vi "Actor Tracker.vi"(8 "error in":errorcluster, 10 "Context":T1, 11 "_Parent Actor Template in":refnum<class "_Parent Actor Template.lvclass">) -> (0 "error out":errorcluster, 3 "_Parent Actor Template out":refnum<class "_Parent Actor Template.lvclass">)   [LabVIEW 2016, in "_Parent Actor Template.lvlib" / "_Parent Actor Template.lvclass"]
uses:
  _Parent Actor Template.lvclass
  Enum - Debug Context.ctl
panel:
  out "Still Running":i32(listbox)
  out "Shutdown\nComplete":bool
  out "Stopped":i32
  out "Started":i32
  out "Shutdown":i32(listbox)
  out "Startup":i32(listbox)
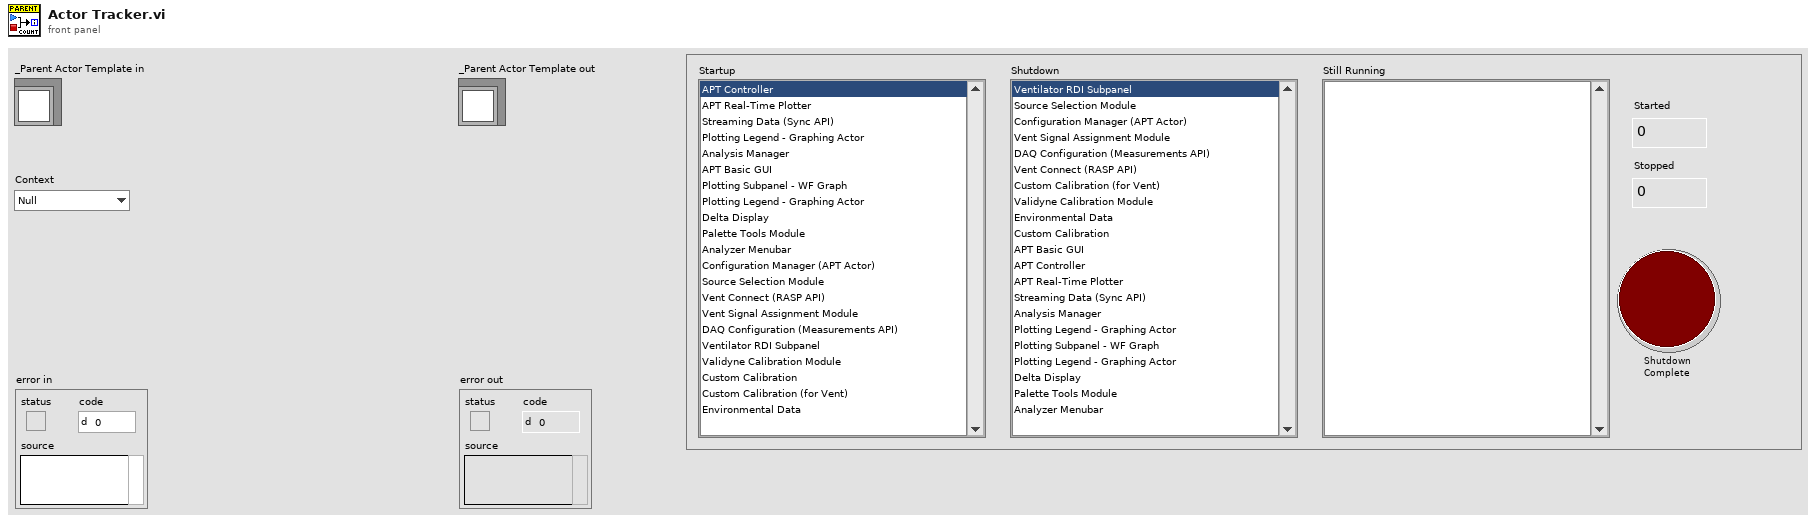
[diagram p1: front panel]
types:
  T1 = typedef "_Parent Actor Template.lvlib/_Parent Actor Template.lvclass/Enum - Debug Context.ctl" = enum16{"Null", "Startup", "Shutdown"}
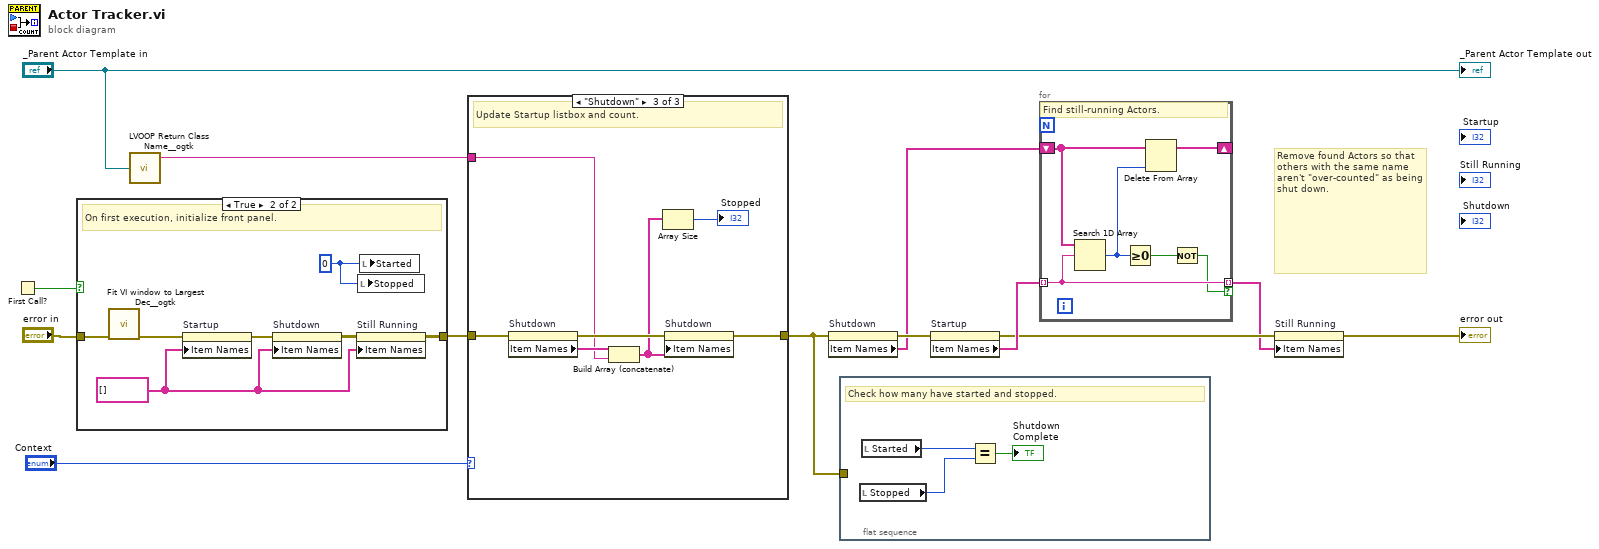
[diagram p0: block diagram]
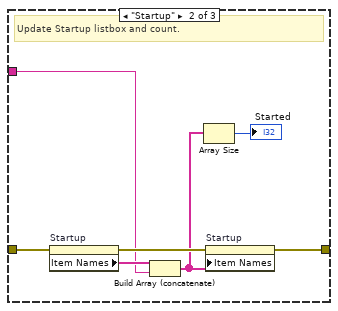
[diagram p3: hidden frame]
diagram:
  # "Remove found Actors so that others with the same name aren't \"over-counted\" as being shut down."
  n1 = First Call?() -> (First Call?: T/F=w12:bool)
  n2 = case shown="True" w12 {
    tunnel: "error in" -> [w14 w21]
    tunnel: [w14 w17] -> w9
    frame False {
    }
    frame True {
      w15 = 0 ("Started")
      w16 = string[] [] ("Item Names")
      # "On first execution, initialize front panel."
      n3 = call <userlib>:"Fit VI window to Largest Dec__ogtk.vi"("error in (no error)"=w21) -> ("error out"=w18:errorcluster)  [unwired: 5 in, 1 out]
      n4 = property on="Startup" class="LstBox (strict)"(error in=w18, "Item Names"=w16) -> (error out=w20:errorcluster)  [unwired: 1 in, 1 out]
      n5 = property on="Shutdown" class="LstBox (strict)"(error in=w20, "Item Names"=w16) -> (error out=w19:errorcluster)  [unwired: 1 in, 1 out]
      n6 = property on="Still Running" class="LstBox (strict)"(error in=w19, "Item Names"=w16) -> (error out=w17:errorcluster)  [unwired: 1 in, 1 out]
      n7 = local write "Stopped"(w15) -> ()
      n8 = local write "Started"(w15) -> ()
    }
  }
  n9 = call <userlib>:"LVOOP Return Class Name__ogtk.vi"("Object"="_Parent Actor Template in") -> ("Class Base Name"=w8:string)  [unwired: 2 out]
  n10 = case shown="\"Shutdown\"" "Context" {
    tunnel: [w22 w27 w34] -> w1
    tunnel: w9 -> [w22 w29 w36]
    tunnel: w8 -> [_ w25 w32]
    frame "Null", Default {
    }
    frame "Startup" {
      # "Update Startup listbox and count."
      n11 = property on="Startup" class="LstBox (strict)"(error in=w29) -> (error out=w28:errorcluster, "Item Names"=w26:string[])  [unwired: 1 in, 1 out]
      n12 = Build Array (concatenate)(w26, w25) -> (w24:string[])
      n13 = Array Size(array=w24) -> (size(s)=→"Started":i32)
      n14 = property on="Startup" class="LstBox (strict)"(error in=w28, "Item Names"=w24) -> (error out=w27:errorcluster)  [unwired: 1 in, 1 out]
    }
    frame "Shutdown" {
      # "Update Startup listbox and count."
      n15 = property on="Shutdown" class="LstBox (strict)"(error in=w36) -> (error out=w35:errorcluster, "Item Names"=w33:string[])  [unwired: 1 in, 1 out]
      n16 = Build Array (concatenate)(w33, w32) -> (w31:string[])
      n17 = Array Size(array=w31) -> (size(s)=→"Stopped":i32)
      n18 = property on="Shutdown" class="LstBox (strict)"(error in=w35, "Item Names"=w31) -> (error out=w34:errorcluster)  [unwired: 1 in, 1 out]
    }
  }
  n19 = property on="Shutdown" class="LstBox (strict)"(error in=w1) -> (error out=w7:errorcluster, "Item Names"=w6:string[])  [unwired: 1 in, 1 out]
  n20 = flat-sequence {
    tunnel: w1 -> [_]
    frame #0 {
      # "Check how many have started and stopped."
      n21 = local read "Stopped"() -> (w38:i32)
      n22 = local read "Started"() -> (w39:i32)
      n23 = Equal?(x=w39, y=w38) -> (x = y?=→"Shutdown\nComplete":bool)
    }
  }
  n24 = property on="Startup" class="LstBox (strict)"(error in=w7) -> (error out=w4:errorcluster, "Item Names"=w5:string[])  [unwired: 1 in, 1 out]
  n25 = for {
    tunnel: w5 -> [w45] mode=indexing
    tunnel: [w45] -> w2 mode=indexing if=w43
    shift-right: [w40] -> _
    shift-left: w6 -> [w42]
    # "Find still-running Actors."
    n26 = Search 1D Array(1D array=w42, element=w45) -> (index of element=w41:i32)  [unwired: 1 in]
    n27 = Greater Or Equal To 0?(x=w41) -> (x >= 0?=w44:bool)
    n28 = Delete From Array(array=w42, index=w41) -> (array with subset deleted=w40:string[])  [unwired: 1 in, 1 out]
    n29 = Not(x=w44) -> (.not. x?=w43:bool)
  }
  n30 = property on="Still Running" class="LstBox (strict)"(error in=w4, "Item Names"=w2) -> (error out=→"error out":errorcluster)  [unwired: 1 in, 1 out]
  "_Parent Actor Template out" <- "_Parent Actor Template in"
